vi "Remove Slave Test Runner.vi"(8 "error in (no error)":errorcluster, 11 "Test Runner in":refnum<class "Test Runner.lvclass">) -> (0 "error out":errorcluster, 3 "Test Runner out":refnum<class "Test Runner.lvclass">)   [LabVIEW 2020, in "Test Runner.lvclass"]
uses:
  Test Runner.lvclass
  Test Runner.lvclass/Test Runner.ctl
  Slave Test Runner/Slave Test Runner.lvclass
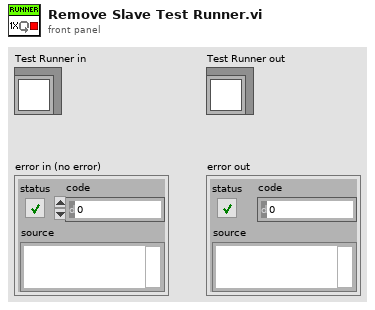
[diagram p1: front panel]
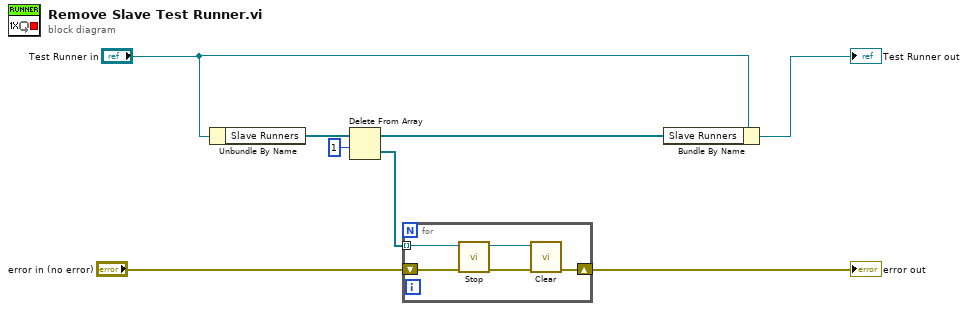
[diagram p0: block diagram]
diagram:
  n1 = Unbundle By Name("Test Runner in") -> ("Slave Runners"=w4:refnum<class "Slave Test Runner.lvclass">[])
  n2 = Delete From Array(array=w4, length=1) -> (deleted portion=w3:refnum<class "Slave Test Runner.lvclass">[], array with subset deleted=w2:refnum<class "Slave Test Runner.lvclass">[])  [unwired: 1 in]
  n3 = for {
    shift-right: [w10] -> w6
    shift-left: "error in (no error)" -> [w13]
    tunnel: w3 -> [w12] mode=indexing
    n4 = call-dynamic "Stop.vi"("error in (no error)"=w13, "Process In"=w12) -> ("error out"=w9:errorcluster, "Process Out"=w11:refnum<class "Slave Test Runner.lvclass">)  [unwired: 7 in, 1 out]
    n5 = call-dynamic "Clear.vi"("error in (no error)"=w9, "Slave Test Runner In"=w11) -> ("error out"=w10:errorcluster)  [unwired: 8 in, 1 out]
  }
  "error out" <- w6
  n6 = Bundle By Name(cluster="Test Runner in", "Slave Runners"=w2) -> (→"Test Runner out":refnum<class "Test Runner.lvclass">)
